vi "F4_discard.vi"(7 "DIscard Channel Info":i32[](array[numeric]), 11 "Array":dbl[][](array[numeric])) -> (3 "array w/ subset deleted":dbl[][](array[numeric]))   [LabVIEW 2014]
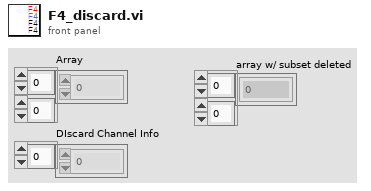
[diagram p1: front panel]
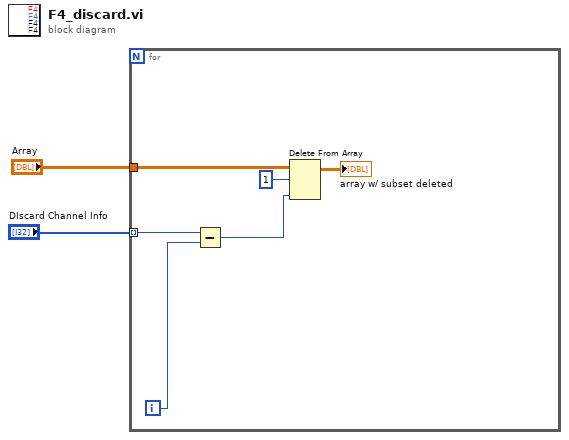
[diagram p0: block diagram]
diagram:
  n1 = for {
    tunnel: "Array" -> [w7]
    tunnel: "DIscard Channel Info" -> [w5] mode=indexing
    i -> [w4]
    n2 = Subtract(x=w5, y=w4) -> (x-y=w3:i32)
    n3 = Delete From Array(array=w7, length=1, index (col)=w3) -> (array with subset deleted=→"array w/ subset deleted":dbl[][])  [unwired: 1 in, 1 out]
  }
